vi "PWM Pulsate.vi"() -> ()   [LabVIEW 2020, in "CTI-Visa-Scratchpad.lvlib"]
uses:
  CTI-Visa-Scratchpad.lvlib
  CTI-Visa/CTI-Visa.lvlib
  <vilib>/ptbypt/NI_PtbyPt.lvlib
panel:
  in  "Speed":i32(slide) scale=1000.0..1.0
  in  "stop":bool
  out "Act. Duty":sgl format="%_6f"
  in  "Port":refnum<visa-resource-name>="COM3"
  in  "Channel":i32
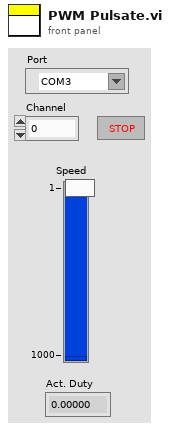
[diagram p1: front panel]
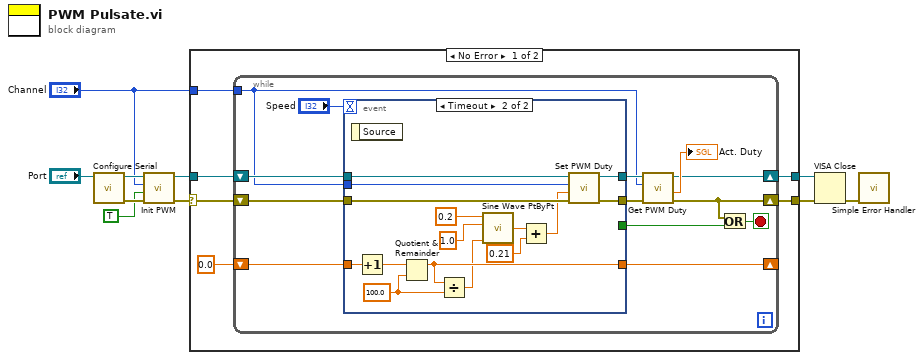
[diagram p0: block diagram]
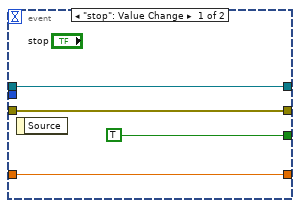
[diagram p2: hidden frame]
diagram:
  n1 = call "Configure Serial.vi"("VISA resource name in"="Port") -> ("error out"=w8:errorcluster, "VISA resource name"=w9:refnum<visa-resource-name>)  [unwired: 9 in]
  n2 = call "Init PWM.vi"("error in (no error)"=w8, "Enable (F)"=TRUE, "Channel"="Channel", "VISA resource name in"=w9) -> ("error out"=w7:errorcluster, "VISA resource name"=w6:refnum<visa-resource-name>)  [unwired: 6 in]
  n3 = case shown="No Error" w7 {
    selector: w7 -> [w15 w49]
    tunnel: w6 -> [w16 w50]
    tunnel: [w14 w50] -> w3
    tunnel: [w13 w49] -> w4
    tunnel: "Channel" -> [w12 _]
    frame No Error {
      n4 = while {
        shift-right: [w20] -> w14
        shift-left: w16 -> [w28]
        shift-right: [w19] -> w13
        shift-left: w15 -> [w27]
        tunnel: w12 -> [w23]
        shift-right: [w17] -> _
        shift-left: 0.0 -> [w18]
        stop <- w29 stop-if-true
        n5 = event shown="[1] Timeout" {
          selector: _ -> [_ _]
          dyn-events: _ -> [_ _]
          timeout: "Speed" -> [_ _]
          tunnel: [w33 w41] -> w25
          tunnel: w28 -> [w33 w46]
          tunnel: [w32 w42] -> w24
          tunnel: w27 -> [w32 w45]
          tunnel: [TRUE _] -> w26
          tunnel: w23 -> [_ w34]
          tunnel: w18 -> [w30 w39]
          tunnel: [w30 w36] -> w17
          event "stop": Value Change {
            n6 = event-data() -> ()  [unwired: 1 in, 1 out]
          }
          event Timeout {
            w37 = 100.0 ("frequency")
            n7 = event-data() -> ()  [unwired: 1 in, 1 out]
            n8 = Increment(x=w39) -> (x+1=w38:dbl)
            n9 = Quotient & Remainder(x=w38, y=w37) -> (x-y*floor(x/y)=w36:dbl)  [unwired: 1 out]
            n10 = Divide(x=w36, y=w37) -> (x/y=w35:dbl)
            n11 = call <vilib>:"Sine Wave PtByPt.vi"("time"=w35, "frequency"=1.0, "amplitude"=0.2) -> ("sine wave"=w44:dbl)  [unwired: 1 in]
            n12 = Add(x=w44, y=0.21) -> (x+y=w40:dbl)
            n13 = call "Set PWM Duty.vi"("error in (no error)"=w45, "Duty % (0-1)"=w40, "Channel"=w34, "VISA resource name in"=w46) -> ("error out"=w42:errorcluster, "VISA resource name"=w41:refnum<visa-resource-name>)  [unwired: 6 in]
          }
        }
        n14 = call "Get PWM Duty.vi"("error in (no error)"=w24, "Channel"=w23, "VISA resource name in"=w25) -> ("error out"=w19:errorcluster, "Duty % (0-1)"=→"Act. Duty":sgl, "VISA resource name"=w20:refnum<visa-resource-name>)  [unwired: 6 in]
        n15 = Or(x=w19, y=w26) -> (x .or. y?=w29:bool)
      }
    }
    frame Error {
    }
  }
  n16 = VISA Close(VISA resource name=w3, error in (no error)=w4) -> (error out=w2:errorcluster)
  n17 = call <vilib>:"Simple Error Handler.vi"("error in (no error)"=w2) -> ()  [unwired: 4 in, 5 out]
